vi "发送数据记录到文档(子VI).vi"(7 "错误输入":errorcluster, 10 "数组":string[](array[string])) -> (0 "错误输出":errorcluster)   [LabVIEW 2016]
uses:
  <vilib>/Utility/sysdir.llb/System Directory Type.ctl
panel:
  out "路径":path
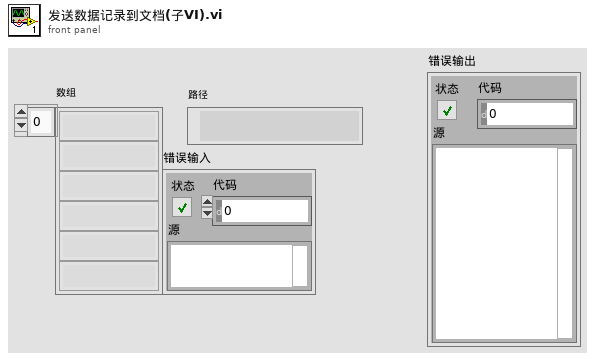
[diagram p1: front panel]
types:
  T1 = typedef "System Directory Type.ctl" = i32
  T2 = enum16{"open", "replace", "create", "open or create", "replace or create", "replace or create with confirmation"}
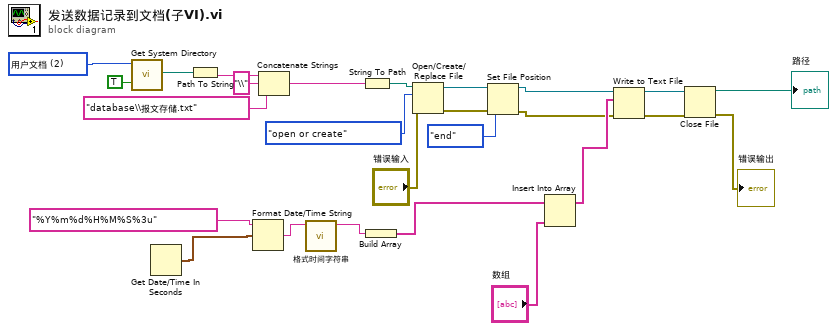
[diagram p0: block diagram]
diagram:
  w17 = T1 2 items=["用户目录"=0, "用户桌面"=1, "用户文档"=2, "用户应用程序数据"=3, "用户设置"=4, "用户临时目录"=5, "公共文档"=6, "公共应用程序数据"=7, "公共设置"=8, "公共缓存"=13, "系统核心库"=9, "系统安装库"=10, "应用程序文件"=11, "启动盘根目录"=12] ("system directory type")
  n1 = call <vilib>:"Get System Directory.vi"("create directory if not found? (F)"=TRUE, "system directory type"=w17) -> ("system directory"=w15:path)  [unwired: 9 in]
  n2 = Get Date/Time In Seconds() -> (seconds since 1Jan1904=w5:timestamp)
  n3 = Path To String(path=w15) -> (string=w14:string)
  n4 = Format Date/Time String(time format string (%c)="%Y%m%d%H%M%S%3u" ("时间格式字符串(%c)"), seconds (now)=w5) -> (date/time string=w3:string)  [unwired: 1 in]
  n5 = Concatenate Strings(w14, "\\" ("字符串"), "database\\报文存储.txt" ("字符串")) -> (w11:string)
  n6 = call "格式时间字符串.vi"("字符串"=w3) -> ("连接的字符串"=w2:string)  [unwired: 10 in]
  n7 = String To Path(string=w11) -> (path=w22:path)
  n8 = Build Array(w2) -> (w1:string[])
  n9 = Open/Create/Replace File(file path (use dialog)=w22, error in="错误输入", operation (0:open)=T2."open or create" ("操作(0:open)")) -> (refnum out=w10:refnum<file>, error out=w9:errorcluster)  [unwired: 3 in, 1 out]
  n10 = Set File Position(refnum=w10, from (0:start)=enum16{"start", "end", "current"}."end" ("自（0:起始）"), error in=w9) -> (refnum out=w8:refnum<file>, error out=w7:errorcluster)  [unwired: 1 in]
  n11 = Insert Into Array(array=w1, new element="数组") -> (w20:string[])  [unwired: 1 in]
  n12 = Write to Text File(file (use dialog)=w8, text=w20, error in=w7) -> (refnum out=w25:refnum<file>, error out=w26:errorcluster)  [unwired: 1 in, 1 out]
  n13 = Close File(refnum=w25, error in=w26) -> (path=→"路径":path, error out=→"错误输出":errorcluster)
